vi "Read Settings.vi"(8 "error in (no error)":errorcluster, 11 "Keithley Source in":refnum<class "Keithley Source.lvclass">) -> (0 "error out":errorcluster, 2 "Settings":string, 3 "Keithley Source out":refnum<class "Keithley Source.lvclass">)   [LabVIEW 2015, in "Keithley Source.lvclass"]
uses:
  Keithley Source.lvclass
  Kethley Source Data.ctl
  OO Devices/Device/Read Controls Snapshot.vi
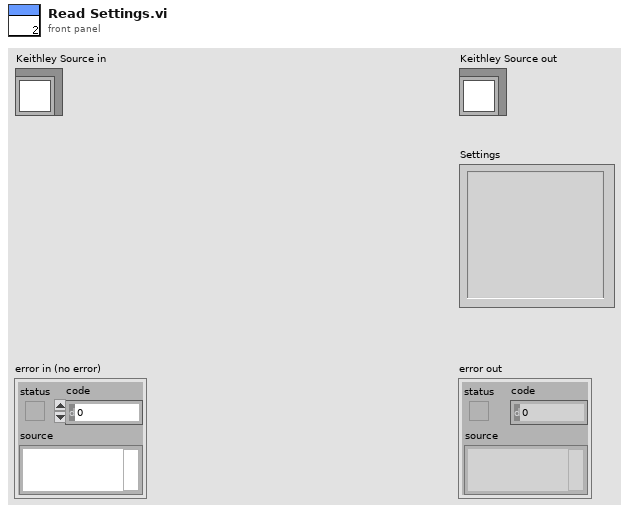
[diagram p1: front panel]
types:
  T1 = typedef "Kethley Source Data.ctl" = cluster{"Mode":enum16{"up-down sweep"}, "Start current":dbl, "End current":dbl, "Current step":dbl, "Compliance":dbl}
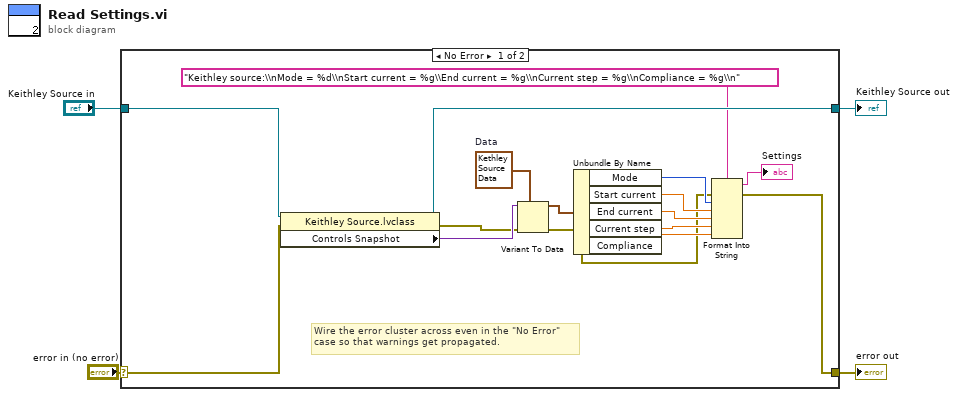
[diagram p0: block diagram]
diagram:
  n1 = case shown="No Error" "error in (no error)" {
    selector: "error in (no error)" -> [w15 w22]
    tunnel: [w5 w22] -> w3
    tunnel: [w16 w21] -> w1
    tunnel: "Keithley Source in" -> [w17 w21]
    frame No Error {
      w19 = T1 {"Mode"=enum."up-down sweep", "Start current"=0.0, "End current"=0.0, "Current step"=0.0, "Compliance"=0.0}  # Data
      # "Wire the error cluster across even in the \"No Error\"\ncase so that warnings get propagated."
      n2 = property class="Keithley Source.lvclass"(reference=w17, error in=w15) -> (reference out=w16:refnum<class "Keithley Source.lvclass">, error out=w18:errorcluster, "Controls Snapshot"=w20:variant)
      n3 = Variant To Data(error in=w18, type=w19, Variant=w20) -> (data=w14:T1, error out=w6:errorcluster)
      n4 = Unbundle By Name(w14) -> ("Mode"=w12:enum16{"up-down sweep"}, "Start current"=w11:dbl, "End current"=w10:dbl, "Current step"=w9:dbl, "Compliance"=w8:dbl)
      n5 = Format Into String(format string="Keithley source:\\nMode = %d\\nStart current = %g\\End current = %g\\nCurrent step = %g\\nCompliance = %g\\n", error in=w6, w12, w11, w10, w9, w8) -> (resulting string=→"Settings":string, error out=w5:errorcluster)  [unwired: 1 in]
    }
    frame Error {
    }
  }
  "error out" <- w3
  "Keithley Source out" <- w1
